vi "Calibration Globals.vi"() -> ()   [LabVIEW 2020]
panel:
  in  "Right ID":string="Right"
  in  "Left ID":string="Left"
  in  "Data folder":path=path "C:/Data"
  in  "Cal Exemplar Folder":path=path "C:/Data/Cal Exemplars"
  in  "Probe Tube Folder":path=path "C:/Data/Probe Tube Calibrations"
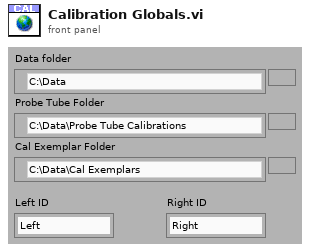
[diagram p1: front panel]
diagram:
